vi "Get Equalization.vi"(2 "acq in":refnum<class "niUSRP Rx DSP v2 FPGA.lvclass">, 11 "ch":u8) -> (4 "equalization":refnum<class "Equalization Interface (IQ 18-bit).lvclass">)   [LabVIEW 2025, in "niUSRP Rx DSP v2 FPGA.lvclass"]
doc: "this VI is an Acquisition class accessor for private data."
uses:
  niUSRP Rx DSP v2 FPGA.lvclass
  <instrlib>/_niInstr/DSP Control/Interface/v1/FPGA/Equalization/IQ 18-bit/Equalization Interface (IQ 18-bit).lvclass
  niUSRP Rx DSP v2 FPGA.lvclass/niUSRP Rx DSP v2 FPGA.ctl
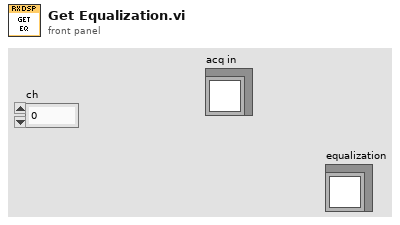
[diagram p1: front panel]
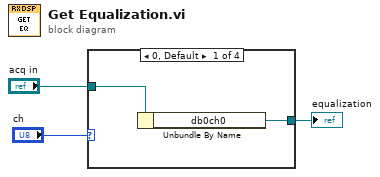
[diagram p0: block diagram]
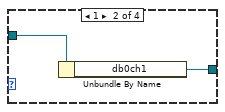
[diagram p2: hidden frame]
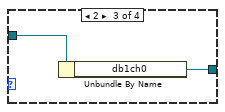
[diagram p3: hidden frame]
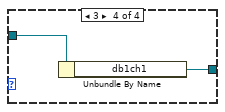
[diagram p4: hidden frame]
diagram:
  n1 = case shown="0, Default" "ch" {
    tunnel: "acq in" -> [w5 w7 w9 w11]
    tunnel: [w4 w6 w8 w10] -> w2
    frame 0, Default {
      n2 = Unbundle By Name(w5) -> ("db0ch0"=w4:refnum<class "Equalization Interface (IQ 18-bit).lvclass">)
    }
    frame 1 {
      n3 = Unbundle By Name(w7) -> ("db0ch1"=w6:refnum<class "Equalization Interface (IQ 18-bit).lvclass">)
    }
    frame 2 {
      n4 = Unbundle By Name(w9) -> ("db1ch0"=w8:refnum<class "Equalization Interface (IQ 18-bit).lvclass">)
    }
    frame 3 {
      n5 = Unbundle By Name(w11) -> ("db1ch1"=w10:refnum<class "Equalization Interface (IQ 18-bit).lvclass">)
    }
  }
  "equalization" <- w2
